vi "WaitforMove.vi"(8 "error in (no error)":errorcluster, 11 "Axis in":refnum<class "Axis.lvclass">) -> (0 "error out":errorcluster, 2 "MoveDone":bool, 3 "Axis out":refnum<class "Axis.lvclass">)   [LabVIEW 2020, in "Axis.lvclass"]
uses:
  Axis.lvclass
  Axis.lvclass/Axis.ctl
  C:/Users/Jonathan/Documents/Clearpath SDK/CSharp Examples/CLRWrapper/x64/Debug/CLRWrapper.dll
  CSharp Examples/CLRWrapper/x64/Debug/CLRWrapper.dll
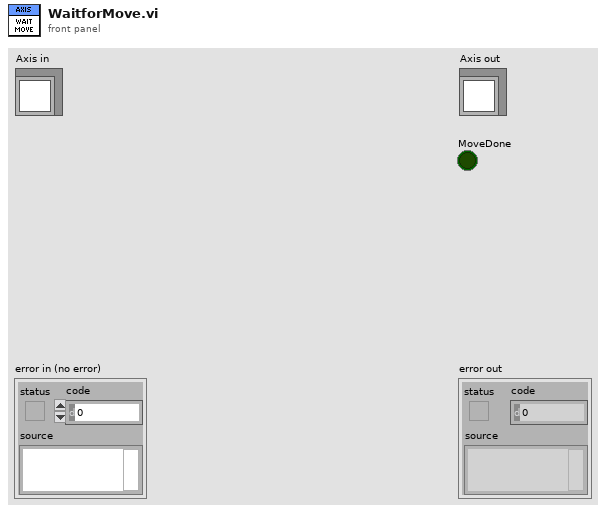
[diagram p1: front panel]
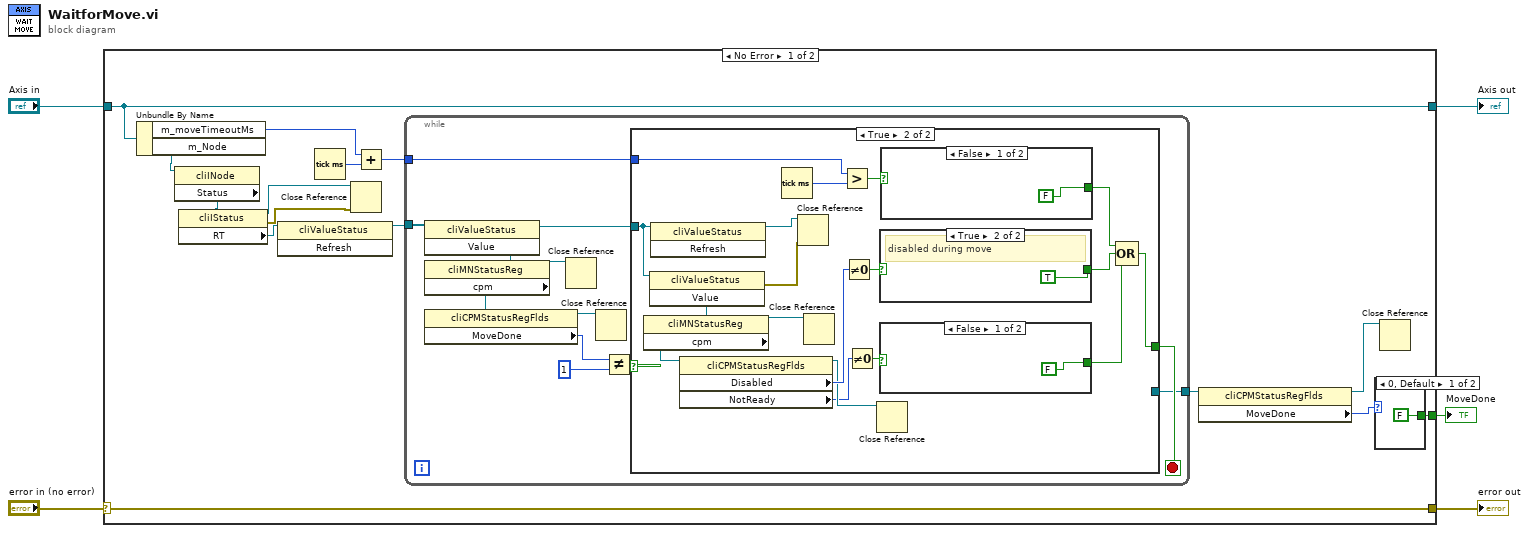
[diagram p0: block diagram]
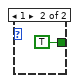
[diagram p2: hidden frame]
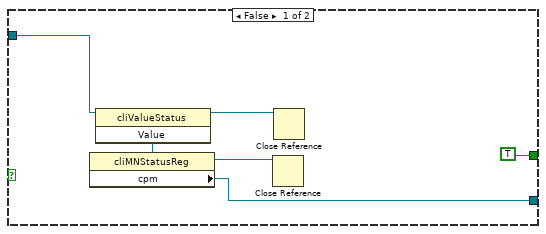
[diagram p3: hidden frame]
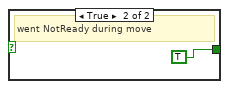
[diagram p4: hidden frame]
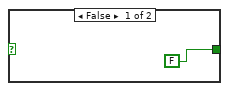
[diagram p5: hidden frame]
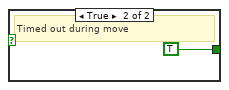
[diagram p6: hidden frame]
diagram:
  n1 = case shown="No Error" "error in (no error)" {
    selector: "error in (no error)" -> [w20 w66]
    tunnel: [w20 w66] -> w4
    tunnel: [w19 w65] -> w2
    tunnel: "Axis in" -> [w19 w65]
    tunnel: [w10 _] -> w1
    frame No Error {
      n2 = Unbundle By Name(w19) -> ("m_moveTimeoutMs"=w11:i32, "m_Node"=w17:refnum<k24>)
      n3 = property class="cliINode"(reference=w17) -> ("Status"=w18:refnum<k24>)  [unwired: 1 in, 2 out]
      n4 = property class="cliIStatus"(reference=w18) -> (reference out=w7:refnum<k24>, error out=w6:errorcluster, "RT"=w16:refnum<k24>)  [unwired: 1 in]
      n5 = invoke class="cliValueStatus" method="Refresh"(reference=w16) -> (reference out=w15:refnum<k24>)  [unwired: 2 in, 2 out]
      n6 = Tick Count (ms)() -> (millisecond timer value=w14:u32)
      n7 = Close Reference(reference=w7, error in (no error)=w6) -> ()  [unwired: 1 out]
      n8 = Add(x=w11, y=w14) -> (x+y=w13:u32)
      n9 = while {
        tunnel: w15 -> [w29]
        tunnel: w13 -> [w32]
        tunnel: [w25] -> w12
        stop <- w33 stop-if-true
        n10 = invoke class="cliValueStatus" method="Value"(reference=w29) -> (reference out=w26:refnum<k24>, "Value"=w31:refnum<k24>)  [unwired: 2 in, 1 out]
        n11 = property class="cliMNStatusReg"(reference=w31) -> (reference out=w24:refnum<k24>, "cpm"=w30:refnum<k24>)  [unwired: 1 in, 1 out]
        n12 = property class="cliCPMStatusRegFlds"(reference=w30) -> (reference out=w23:refnum<k24>, "MoveDone"=w28:u16)  [unwired: 1 in, 1 out]
        n13 = Close Reference(reference=w24) -> ()  [unwired: 1 in, 1 out]
        n14 = Close Reference(reference=w23) -> ()  [unwired: 1 in, 1 out]
        n15 = Not Equal?(x=w28, y=u16 1) -> (x != y?=w34:bool)
        n16 = case shown="True" w34 {
          tunnel: [TRUE w55] -> w33
          tunnel: w32 -> [_ w52]
          tunnel: w26 -> [w38 w50]
          tunnel: [w37 _] -> w25
          frame False {
            n17 = invoke class="cliValueStatus" method="Value"(reference=w38) -> (reference out=w36:refnum<k24>, "Value"=w39:refnum<k24>)  [unwired: 2 in, 1 out]
            n18 = property class="cliMNStatusReg"(reference=w39) -> (reference out=w35:refnum<k24>, "cpm"=w37:refnum<k24>)  [unwired: 1 in, 1 out]
            n19 = Close Reference(reference=w35) -> ()  [unwired: 1 in, 1 out]
            n20 = Close Reference(reference=w36) -> ()  [unwired: 1 in, 1 out]
          }
          frame True {
            n21 = invoke class="cliValueStatus" method="Value"(reference=w50) -> (error out=w41:errorcluster, "Value"=w51:refnum<k24>)  [unwired: 2 in, 1 out]
            n22 = property class="cliMNStatusReg"(reference=w51) -> (reference out=w44:refnum<k24>, "cpm"=w49:refnum<k24>)  [unwired: 1 in, 1 out]
            n23 = invoke class="cliValueStatus" method="Refresh"(reference=w50) -> (reference out=w45:refnum<k24>)  [unwired: 2 in, 2 out]
            n24 = property class="cliCPMStatusRegFlds"(reference=w49) -> (reference out=w43:refnum<k24>, "Disabled"=w47:u16, "NotReady"=w42:u16)  [unwired: 1 in, 1 out]
            n25 = Tick Count (ms)() -> (millisecond timer value=w54:u32)
            n26 = Close Reference(reference=w45, error in (no error)=w41) -> ()  [unwired: 1 out]
            n27 = Close Reference(reference=w44) -> ()  [unwired: 1 in, 1 out]
            n28 = Greater?(x=w52, y=w54) -> (0:w53:bool)
            n29 = Not Equal To 0?(x=w47) -> (x != 0?=w48:bool)
            n30 = Not Equal To 0?(x=w42) -> (x != 0?=w46:bool)
            n31 = Close Reference(reference=w43) -> ()  [unwired: 1 in, 1 out]
            n32 = case shown="True" w48 {
              tunnel: [FALSE TRUE] -> w58
              frame False {
              }
              frame True {
                # "disabled during move"
              }
            }
            n33 = case shown="False" w46 {
              tunnel: [FALSE TRUE] -> w57
              frame False {
              }
              frame True {
                # "went NotReady during move"
              }
            }
            n34 = case shown="False" w53 {
              tunnel: [FALSE TRUE] -> w56
              frame False {
              }
              frame True {
                # "Timed out during move"
              }
            }
            n35 = Compound Arithmetic op=OR(w56, w58, w57) -> (w55:bool)
          }
        }
      }
      n36 = property class="cliCPMStatusRegFlds"(reference=w12) -> (reference out=w8:refnum<k24>, "MoveDone"=w9:u16)  [unwired: 1 in, 1 out]
      n37 = case shown="0, Default" w9 {
        tunnel: [FALSE TRUE] -> w10
        frame 0, Default {
        }
        frame 1 {
        }
      }
      n38 = Close Reference(reference=w8) -> ()  [unwired: 1 in, 1 out]
    }
    frame Error {
    }
  }
  "error out" <- w4
  "Axis out" <- w2
  "MoveDone" <- w1
